vi "Forward Scale.vi"() -> ()   [LabVIEW 2017]
uses:
  Support Code/Starting Position.ctl
  <vilib>/Rock Robotics/WPI/Framework/Command Status Info.ctl
  <vilib>/Rock Robotics/WPI/Framework/Completion Status.ctl
  <vilib>/Rock Robotics/WPI/Framework/Completion Notifier.ctl
panel:
  out "Command Info Out":T1
  in  "Dist. to Scale":dbl
  in  "Turn Target Angle":dbl
  in  "Target Angle":dbl
  in  "Distance":dbl
  in  "Command Info In":T1
  in  "Starting Position":T4=enum."Far Right"
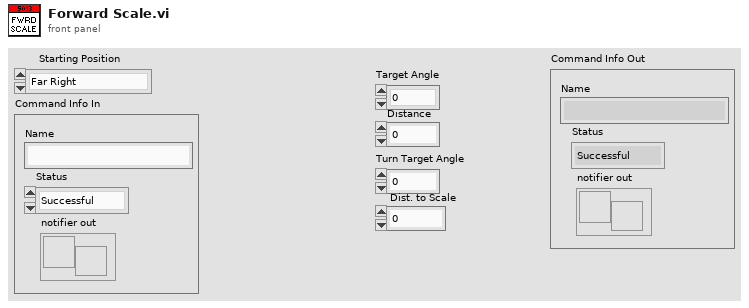
[diagram p1: front panel]
types:
  T1 = typedef "Command Status Info.ctl" = cluster{"Name":string, "Status":T2, "notifier out":T3}
  T2 = typedef "Completion Status.ctl" = enum16{"Successful", "Aborted", "Incomplete"}
  T3 = typedef "Completion Notifier.ctl" = refnum<notifier>
  T4 = typedef "Starting Position.ctl" = enum16{"Left", "Far Left", "Center", "Right", "Far Right"}
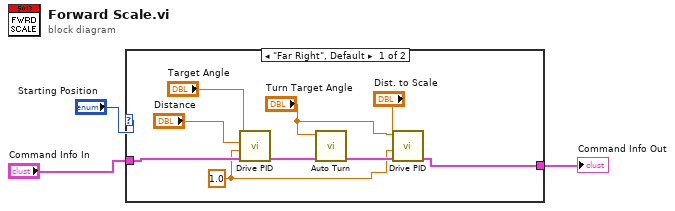
[diagram p0: block diagram]
diagram:
  n1 = case shown="\"Far Right\", Default" "Starting Position" {
    tunnel: "Command Info In" -> [w11 w13]
    tunnel: [w4 w13] -> w1
    frame "Far Right", Default {
      w9 = 1.0 ("Speed")
      n2 = call "Drive PID.vi"("Command Info In"=w11, "Speed"=w9, "Distance"="Distance", "Target Angle"="Target Angle") -> ("Command Info Out"=w12:T1)  [unwired: 7 in]
      n3 = call "Auto Turn.vi"("Command Info In"=w12, "Target Angle"="Turn Target Angle") -> ("Command Info Out"=w10:T1)  [unwired: 9 in]
      n4 = call "Drive PID.vi"("Command Info In"=w10, "Speed"=w9, "Distance"="Dist. to Scale", "Target Angle"="Turn Target Angle") -> ("Command Info Out"=w4:T1)  [unwired: 7 in]
    }
    frame "Far Left" {
    }
  }
  "Command Info Out" <- w1
